vi "IMAQ-MWT GALVO XY Calibration (HOST).vi"() -> ()   [LabVIEW 2017]
uses:
  Modules/Common/Controls (HOST)/Image Size.ctl
  Modules/Common/Controls (HOST)/REF.ctl
  Modules/Common/Controls (HOST)/Image Queue Bundle.ctl
  Modules/Common/Controls (HOST)/Data to Disk Bundle.ctl
  Modules/Common/Controls (HOST)/File Name Prefix.ctl
  Modules/Common/Controls (HOST)/FPGA REF (MWT).ctl
  Modules/Common/Controls (HOST)/Experiment Mode.ctl
  Modules/Common/Controls (HOST)/Main States.ctl
  Modules/Common/Controls (HOST)/IMAQ Parameters.ctl
  Modules/Common/Controls (HOST)/File REF.ctl
  <vilib>/vision/Avi.llb/IMAQ AVI2 Refnum.ctl
  <vilib>/DAQmx/write.llb/DAQmx Write (Analog 1D DBL NChan 1Samp).vi
  <vilib>/Utility/error.llb/Error Cluster From Error Code.vi
  <vilib>/rvi/errors/niLvFpgaAdjustHostInterfaceError.vi
  <vilib>/FPGAPlugInAG/Dynamic/niLvFpga_Close_Dynamic.vi
  <vilib>/DAQmx/configure/timing.llb/DAQmx Timing (Sample Clock).vi
  <vilib>/DAQmx/miscellaneous.llb/DAQmx Fill In Error Info.vi
  <vilib>/rvi/interface/nirviReadWriteControl/nirviReadWriteControl.xnode
  <vilib>/rvi/interface/nirviCloseFPGA/nirviCloseFPGA.xnode
  NiFpgaLv.dll
  <vilib>/rvi/interface/Simulation/niFpgaSimulationCallBeginRW.vi
  <vilib>/vision/NI_Vision_Development_Module.lvlib
  <vilib>/Utility/file.llb/Write Delimited Spreadsheet (I64).vi
panel:
  in  "Calibrate":bool
  in  "Stop Button":bool
  out "GALVO Voltage":cluster{"X":dbl, "Y ":dbl}[](array[cluster]) {"X" format="%.3f"; "Y" format="%.3f"}
  out "Scan spots":cluster{"X":i32, "Y":i32}[](array[cluster])=[{"X"=200, "Y"=200}, {"X"=3000, "Y"=200}]
  in  "DAQmx Task Name":refnum<k21>="GALVO"
  out "IR SPOT (Measured)":cluster{"X":i32, "Y":i32}
  in  "Tab Control":enum32{"Setup"}(tab)
  in  "Image Size":T1={"Height"=3072, "Width"=3200}
  in  "Experiment Mode":T2
  in  "Pixel Intensity Range":cluster{"Low":u8, "High":u8}={"Low"=25, "High"=135}
  in  "Exp. Time (S)":dbl=120.0
  in  "Go":bool
  in  "Subtract BG":bool=TRUE
  in  "Replay Interval (ms)":u32=1000
  in  "Swap Bytes":bool
  out "Particle Reports (Pixels)":T3(array[cluster]) {"Orientation" format="%.2f"; "Dimensions"."Height" format="%.2f"; "Dimensions"."Width" format="%.2f"; "Center of Mass"."Y" format="%.2f"; "Center of Mass"."X" format="%.2f"; "Bounding Rect"."Bottom" format="%.2f"; "Bounding Rect"."Right" format="%.2f"; "Bounding Rect"."Top" format="%.2f"; "Bounding Rect"."Left" format="%.2f"; "Number of Holes" format="%.2f"; "Area" format="%.2f"}
  in  "Range":cluster{"Low":sgl, "High":sgl}={"Low"=3.0, "High"=255.0}
  in  "Selection Values":T5(array[cluster])=[{"Measurement Parameter"=18, "Range Lower Value"=50.0, "Range Upper Value"=1000.0, "Range"=FALSE, "Measurement Type"=FALSE}] {"Measurement Parameter" items=["Center of Mass X", "Center of Mass Y", "First Pixel X", "First Pixel Y", "Bounding Rect Left", "Bounding Rect Top", "Bounding Rect Right", "Bounding Rect Bottom", "Max Feret Diameter Start X", "Max Feret Diameter Start Y", "Max Feret Diameter End X", "Max Feret Diameter End Y", "Max Horiz. Segment Length Left", "Max Horiz. Segment Length Right", "Max Horiz. Segment Length Row", "-", "Bounding Rect Width", "Bounding Rect Height", "Bounding Rect Diagonal", "Perimeter", "Convex Hull Perimeter", "Holes' Perimeter", "Max Feret Diameter", "Equivalent Ellipse Major Axis", "Equivalent Ellipse Minor Axis", "Equivalent Ellipse Minor Axis (Feret)", "Equivalent Rect Long Side", "Equivalent Rect Short Side", "Equivalent Rect Diagonal", "Equivalent Rect Short Side (Feret)", "Average Horiz. Segment Length", "Average Vert. Segment Length", "Hydraulic Radius", "Waddel Disk Diameter", "-", "Area", "Holes' Area", "Particle & Holes' Area", "Convex Hull Area", "Image Area", "-", "Number of Holes", "Number of Horiz. Segments", "Number of Vert. Segments", "-", "Orientation", "Max Feret Diameter Orientation", "-", "% Area/Image Area", "% Area/(Particle & Holes' Area)", "Ratio of Equivalent Ellipse Axes", "Ratio of Equivalent Rect Sides", "-", "Elongation Factor", "Compactness Factor", "Heywood Circularity Factor", "Type Factor", "-", "Sum X", "Sum Y", "Sum XX", "Sum XY", "Sum YY", "Sum XXX", "Sum XXY", "Sum XYY", "Sum YYY", "-", "Moment of Inertia XX", "Moment of Inertia XY", "Moment of Inertia YY", "Moment of Inertia XXX", "Moment of Inertia XXY", "Moment of Inertia XYY", "Moment of Inertia YYY", "Norm. Moment of Inertia XX", "Norm. Moment of Inertia XY", "Norm. Moment of Inertia YY", "Norm. Moment of Inertia XXX", "Norm. Moment of Inertia XXY", "Norm. Moment of Inertia XYY", "Norm. Moment of Inertia YYY", "Hu Moment 1", "Hu Moment 2", "Hu Moment 3", "Hu Moment 4", "Hu Moment 5", "Hu Moment 6", "Hu Moment 7"]; "Range Lower Value" format="%.2f"; "Range Upper Value" format="%.2f"}
  out "Number of Particles":i32
  out "Frame #":u32
  out "Frame Rate":u32
  in  "GALVO Input Voltage (V)":T6 {"GALVO 4"."Y" format="%.3f"; "GALVO 4"."X" format="%.3f"; "GALVO 3"."Y" format="%.3f"; "GALVO 3"."X" format="%.3f"; "GALVO 2"."Y" format="%.3f"; "GALVO 2"."X" format="%.3f"; "GALVO 1"."Y" format="%.3f"; "GALVO 1"."X" format="%.3f"}
  in  "Start Location (Pixels)":cluster{"X":i32, "Y":i32}={"X"=300, "Y"=300}
  in  "End Location (Pixels)":cluster{"X":i32, "Y":i32}={"X"=2800, "Y"=2800}
  in  "STEP Size (Pixels)":i32=50
  in  "Y Reverse":bool=TRUE
  in  "X Reverse":bool
  in  "GALVO #":T7(ring)
  out "Elapsed Time (s)":dbl format="%.1f"
  out "Exp. Status":string="Camera Connected"
  out "REF":T8
  out "Command Q":refnum<queue>
  out "Display":T11(plugin-control)
  out "Stopped?":bool
  # "GALVO XY Auto Calibration"
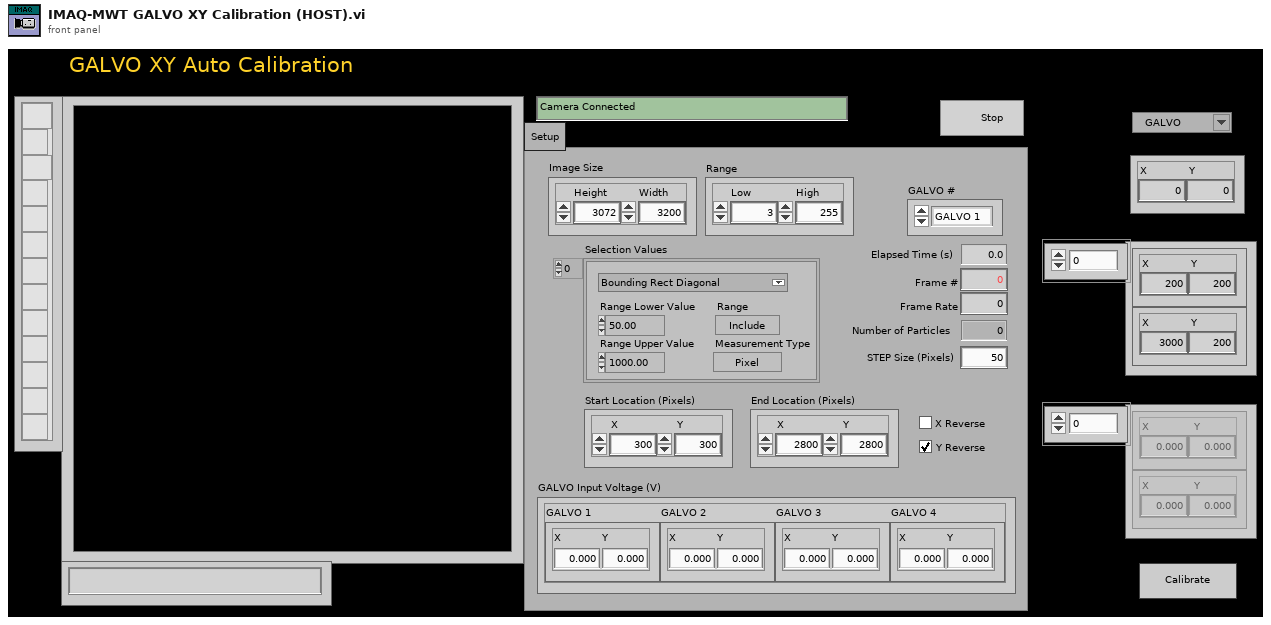
[diagram p1: front panel]
types:
  T1 = typedef "Image Size.ctl" = cluster{"Height":u16, "Width":u16}
  T2 = typedef "Experiment Mode.ctl" = enum16{"Live", "Replay"}
  T3 = cluster{"Area":dbl, "Number of Holes":dbl, "Bounding Rect":cluster{"Left":dbl, "Top":dbl, "Right":dbl, "Bottom":dbl}, "Center of Mass":cluster{"X":dbl, "Y":dbl}, "Orientation":dbl, "Dimensions":cluster{"Width":dbl, "Height":dbl}}[]
  T4 = typedef "Particle Parameters" = i32
  T5 = cluster{"Measurement Parameter":T4, "Range Lower Value":dbl, "Range Upper Value":dbl, "Range":bool, "Measurement Type":bool}[]
  T6 = cluster{"GALVO 1":cluster{"X":dbl, "Y ":dbl}, "GALVO 2":cluster{"X":dbl, "Y ":dbl}, "GALVO 3":cluster{"X":dbl, "Y ":dbl}, "GALVO 4":cluster{"X":dbl, "Y ":dbl}}
  T7 = enum16{"GALVO 1", "GALVO 2", "GALVO 3", "GALVO 4"}
  T8 = typedef "REF.ctl" = cluster{"Queue REF":T9, "FPGA REF (MWT)":T10}
  T9 = typedef "Image Queue Bundle.ctl" = cluster{"Disk Image":refnum<queue>, "Image Blocks":refnum<queue>, "Display Image":refnum<queue>, "BG Image":refnum<queue>, "Tag Image":refnum<queue>, "DLL Input":refnum<queue>, "DMD Input":refnum<queue>, "GALVO Input":refnum<queue>}
  T10 = typedef "FPGA REF (MWT).ctl" = refnum<k20>
  T11 = typedef "IMAQ Image.ctl" = refnum<image>
  T12 = enum8{"Enabled", "Disabled", "Disabled and Grayed Out"}
  T13 = typedef "Main States.ctl" = enum16{"Open FPGA", "Initialize", "Preview", "Acquire Images", "STOP"}
  T14 = typedef "IMAQ Parameters.ctl" = cluster{"File REF":T15, "Frame Data":cluster{"Width":u32, "Height":u32, "Frames Per Second":u32, "Codec":string}, "File Type":string, "Experiment Mode":T2, "Movie File Path":path}
  T15 = typedef "File REF.ctl" = cluster{"AVI REF":T16, "DBDE REF":refnum<file>}
  T16 = typedef "IMAQ AVI2 Refnum.ctl" = refnum<k20>
  T17 = typedef "Data to Disk Bundle.ctl" = cluster{"Frame Number":u64, "Time Stamp (us)":u64, "Image Data":u64[], "Contour":u32[], "Raw Image REF":refnum<data-value>, "Block Image REF":refnum<data-value>, "Block Box":u64[], "SPINE":u32[], "HT Angle":u64[], "Block Position":u64[], "SPINE Count":u32[], "Contour Count":u32[], "SPINE DIR":u8[]}
  T18 = cluster{"Area":dbl, "Number of Holes":dbl, "Bounding Rect":cluster{"Left":dbl, "Top":dbl, "Right":dbl, "Bottom":dbl}, "Center of Mass":cluster{"X":dbl, "Y":dbl}, "Orientation":dbl, "Dimensions":cluster{"Width":dbl, "Height":dbl}}
  T19 = cluster{"Left":dbl, "Top":dbl, "Right":dbl, "Bottom":dbl}
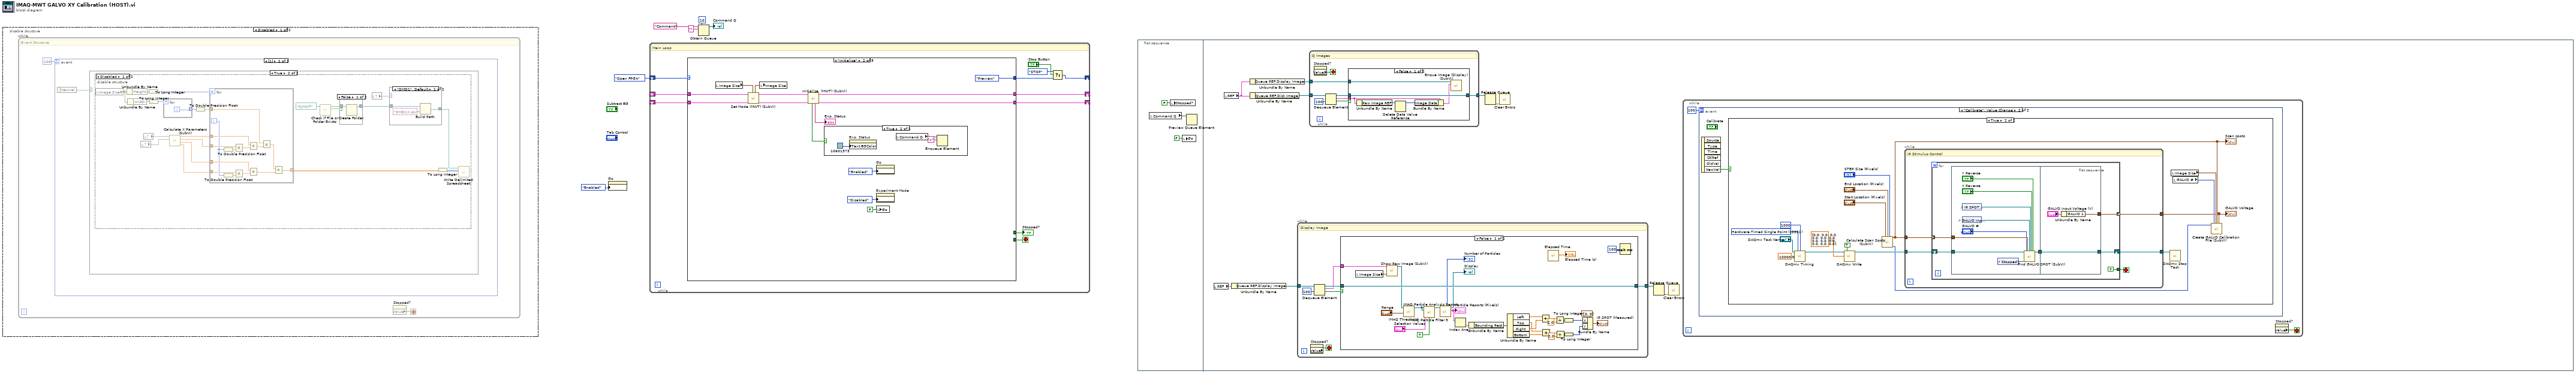
[diagram p0: block diagram]
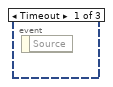
[diagram p2: hidden frame]
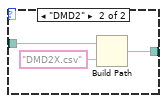
[diagram p5: hidden frame]
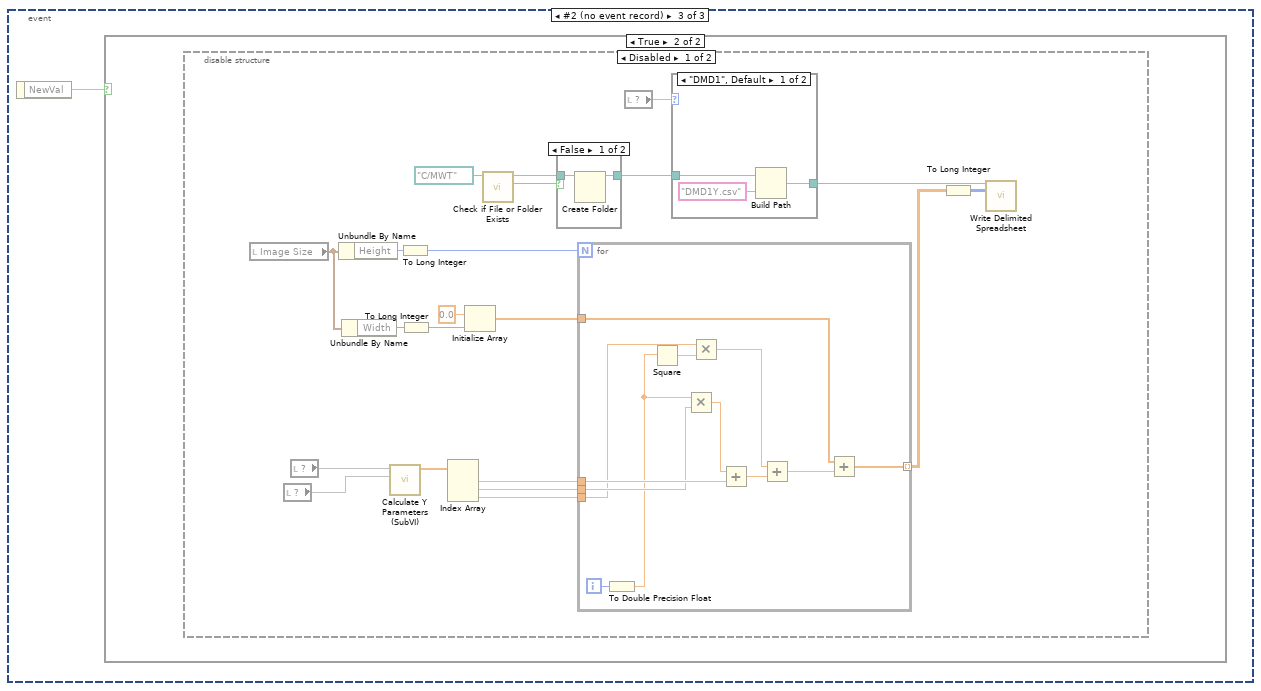
[diagram p7: hidden frame]
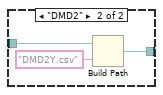
[diagram p10: hidden frame]
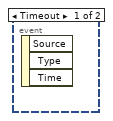
[diagram p13: hidden frame]
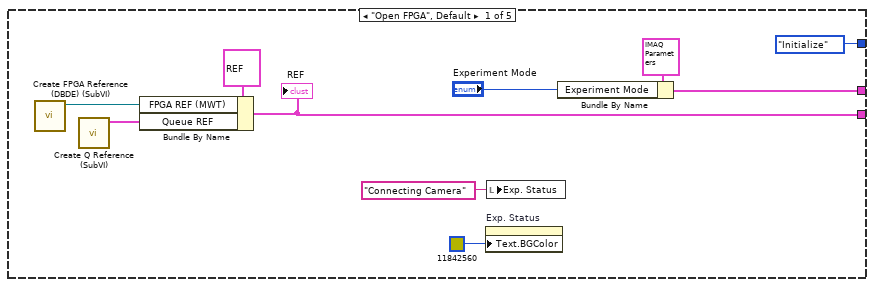
[diagram p17: hidden frame]
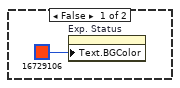
[diagram p18: hidden frame]
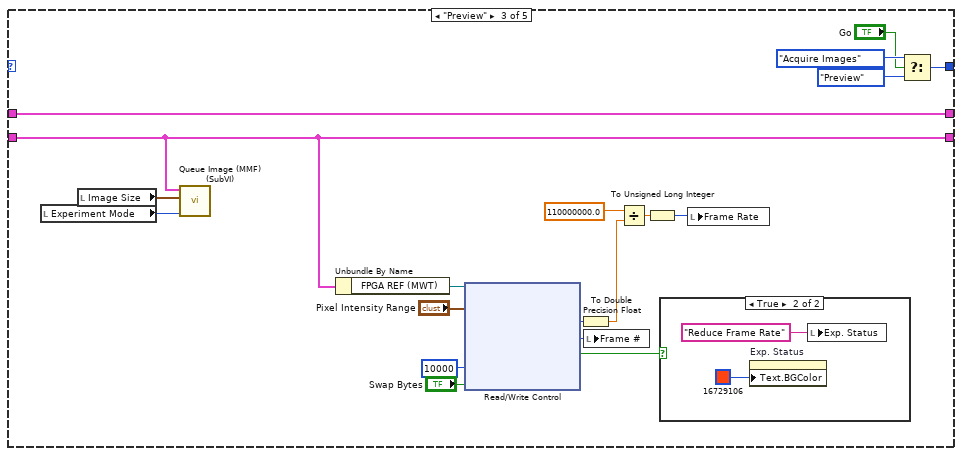
[diagram p19: hidden frame]
diagram:
  n1 = disable-structure shown="Disabled" {
    frame Disabled {
      n2 = while {
        stop <- w8 stop-if-true
        # "Event Structure"
        n3 = event shown="[1]" {
          selector: _ -> [_ _ _]
          dyn-events: _ -> [_ _ _]
          timeout: 100 -> [_ _ _]
          event Timeout {
            n4 = event-data() -> ()  [unwired: 1 in, 1 out]
          }
          event #1 (no event record) {
            n5 = event-data() -> ("NewVal"=w9)  [unwired: 1 in]
            n6 = case shown="True" w9 {
              frame False {
              }
              frame True {
                n7 = disable-structure shown="Disabled" {
                  frame Disabled {
                    n8 = local read "Image Size"() -> (w18:T1)
                    n9 = Unbundle By Name(w18) -> ("Height"=w30:u16)
                    n10 = Unbundle By Name(w18) -> ("Width"=w28:u16)
                    n11 = local read item#-1() -> (w24)
                    n12 = local read item#-1() -> (w23)
                    n13 = To Long Integer(number=w30) -> (32bit integer=w29:i32)
                    n14 = To Long Integer(number=w28) -> (32bit integer=w27:i32)
                    n15 = for {
                      N: w27 -> [_]
                      tunnel: [w40] -> w26 mode=indexing
                      i -> [w40]
                    }
                    n16 = call "Calculate X Parameters (SubVI).vi"("Camera"=w24, "DMD"=w23) -> ("Intercept Rate"=w19:dbl, "Intercept"=w20:dbl, "Slope Rate"=w21:dbl, "Slope"=w22:dbl)  [unwired: 6 in]
                    n17 = To Double Precision Float(number=w26) -> (double precision float=w25:dbl[])
                    n18 = for {
                      N: w29 -> [_]
                      tunnel: w25 -> [w49]
                      tunnel: w22 -> [w51]
                      tunnel: w21 -> [w54]
                      tunnel: w20 -> [w48]
                      tunnel: w19 -> [w45]
                      tunnel: [w41] -> w17 mode=indexing
                      i -> [w44]
                      n19 = To Double Precision Float(number=w44) -> (double precision float=w53:dbl)
                      n20 = To Double Precision Float(number=w44) -> (double precision float=w46:dbl)
                      n21 = Multiply(x=w54, y=w53) -> (x*y=w52:dbl)
                      n22 = Multiply(x=w45, y=w46) -> (x*y=w47:dbl)
                      n23 = Add(x=w51, y=w52) -> (x+y=w50:dbl)
                      n24 = Add(x=w48, y=w47) -> (x+y=w43:dbl)
                      n25 = Multiply(x=w49, y=w50) -> (x*y=w42:dbl[])
                      n26 = Add(x=w42, y=w43) -> (x+y=w41:dbl[])
                    }
                    n27 = call <vilib>:"Check if File or Folder Exists.vi"("path"=path "C:/MWT") -> ("file or folder exists?"=w14:bool, "dup path"=w13:path)  [unwired: 8 in, 1 out]
                    n28 = case shown="False" w14 {
                      tunnel: w13 -> [w32 w33]
                      tunnel: [w31 w33] -> w12
                      frame False {
                        n29 = Create Folder(path (use dialog)=w32) -> (created path=w31:path)  [unwired: 2 in, 2 out]
                      }
                      frame True {
                      }
                    }
                    n30 = local read item#-1() -> (w16)
                    n31 = case shown="\"DMD1\", Default" w16 {
                      tunnel: w12 -> [w36 w39]
                      tunnel: [w34 w37] -> w11
                      frame "DMD1", Default {
                        n32 = Build Path(base path=w36, name or relative path="DMD1X.csv") -> (appended path=w34:path)
                      }
                      frame "DMD2" {
                        n33 = Build Path(base path=w39, name or relative path="DMD2X.csv") -> (appended path=w37:path)
                      }
                    }
                    n34 = To Long Integer(number=w17) -> (32bit integer=w10:i32[][])
                    n35 = call-poly <vilib>:"Write Delimited Spreadsheet.vi"("file path (dialog if empty)"=w11, "2D data"=w10) -> ()  [unwired: 12 in, 2 out]
                  }
                  frame Enabled {
                  }
                }
              }
            }
          }
          event #2 (no event record) {
            n36 = event-data() -> ("NewVal"=w55)  [unwired: 1 in]
            n37 = case shown="True" w55 {
              frame False {
              }
              frame True {
                n38 = disable-structure shown="Disabled" {
                  frame Disabled {
                    n39 = local read "Image Size"() -> (w70:T1)
                    n40 = local read item#-1() -> (w74)
                    n41 = local read item#-1() -> (w75)
                    n42 = Unbundle By Name(w70) -> ("Height"=w71:u16)
                    n43 = Unbundle By Name(w70) -> ("Width"=w73:u16)
                    n44 = call "Calculate Y Parameters (SubVI).vi"("Camera"=w74, "DMD"=w75) -> ("Polynomial Coefficients"=w76:dbl[])  [unwired: 9 in]
                    n45 = To Long Integer(number=w71) -> (32bit integer=w72:i32)
                    n46 = To Long Integer(number=w73) -> (32bit integer=w59:i32)
                    n47 = Index Array(array=w76) -> (element #1=w61:dbl, element #2=w60:dbl, element #3=w56:dbl)  [unwired: 3 in]
                    n48 = Initialize Array(0.0 ("element"), w59) -> (w57:dbl[])
                    n49 = call <vilib>:"Check if File or Folder Exists.vi"("path"=path "C:/MWT") -> ("file or folder exists?"=w66:bool, "dup path"=w65:path)  [unwired: 8 in, 1 out]
                    n50 = case shown="False" w66 {
                      tunnel: w65 -> [w78 w79]
                      tunnel: [w77 w79] -> w64
                      frame False {
                        n51 = Create Folder(path (use dialog)=w78) -> (created path=w77:path)  [unwired: 2 in, 2 out]
                      }
                      frame True {
                      }
                    }
                    n52 = for {
                      N: w72 -> [_]
                      tunnel: [w87] -> w69 mode=indexing
                      tunnel: w61 -> [w95]
                      tunnel: w60 -> [w94]
                      tunnel: w57 -> [w86]
                      tunnel: w56 -> [w90]
                      i -> [w93]
                      n53 = To Double Precision Float(number=w93) -> (double precision float=w92:dbl)
                      n54 = Square(x=w92) -> (x^2=w91:dbl)
                      n55 = Multiply(x=w92, y=w94) -> (x*y=w97:dbl)
                      n56 = Multiply(x=w90, y=w91) -> (x*y=w88:dbl)
                      n57 = Add(x=w97, y=w95) -> (x+y=w96:dbl)
                      n58 = Add(x=w88, y=w96) -> (x+y=w89:dbl)
                      n59 = Add(x=w86, y=w89) -> (x+y=w87:dbl[])
                    }
                    n60 = local read item#-1() -> (w68)
                    n61 = case shown="\"DMD1\", Default" w68 {
                      tunnel: w64 -> [w80 w83]
                      tunnel: [w82 w85] -> w63
                      frame "DMD1", Default {
                        n62 = Build Path(base path=w80, name or relative path="DMD1Y.csv") -> (appended path=w82:path)
                      }
                      frame "DMD2" {
                        n63 = Build Path(base path=w83, name or relative path="DMD2Y.csv") -> (appended path=w85:path)
                      }
                    }
                    n64 = To Long Integer(number=w69) -> (32bit integer=w62:i32[][])
                    n65 = call-poly <vilib>:"Write Delimited Spreadsheet.vi"("file path (dialog if empty)"=w63, "2D data"=w62) -> ()  [unwired: 12 in, 2 out]
                  }
                  frame Enabled {
                  }
                }
              }
            }
          }
        }
        n66 = property on="Stopped?" class="Bool (strict)"() -> ("Value"=w8:bool)  [unwired: 2 in, 2 out]
      }
    }
    frame Enabled {
    }
  }
  n67 = property on="Go" class="Bool (strict)"("DisabledEnum"=T12."Enabled" ("Disabled")) -> ()  [unwired: 2 in, 2 out]
  n68 = while {
    shift-right: [w107] -> _
    shift-left: _ -> [w106]
    shift-right: [w98] -> _
    shift-left: Main_States."Open FPGA" -> [w108]
    shift-right: [w100] -> _
    shift-left: _ -> [w99]
    stop <- w104 stop-if-true
    # "Main Loop"
    n69 = case shown="\"Initialize\"" w108 {
      tunnel: [w115 w119 w140 w163 w193] -> w107
      tunnel: w106 -> [_ w120 w140 w163 w193]
      tunnel: [Main_States."Initialize" Main_States."Preview" w154 w182 Main_States."STOP"] -> w105
      tunnel: [_ _ _ _ w195] -> w104
      tunnel: [_ _ _ _ w195] -> w103
      tunnel: [w109 w124 w147 w166 w192] -> w100
      tunnel: w99 -> [_ w131 w147 w166 w192]
      frame "Open FPGA", Default {
        n70 = call "Create FPGA Reference (DBDE) (SubVI).vi"() -> ("FPGA REF (MWT)"=w117:T10)  [unwired: 11 in]
        n71 = call "Create Q Reference (SubVI).vi"() -> ("Image Queue"=w116:T9)  [unwired: 11 in]
        n72 = Bundle By Name(cluster=T8 {"Queue REF"={"Disk Image"=refnum, "Image Blocks"=refnum, "Display Image"=refnum, "BG Image"=refnum, "Tag Image"=refnum, "DLL Input"=refnum, "DMD Input"=refnum, "GALVO Input"=refnum}, "FPGA REF (MWT)"=refnum}, "FPGA REF (MWT)"=w117, "Queue REF"=w116) -> (w115:T8)
        "REF" <- w115
        n73 = property on="Exp. Status" class="Str"("Text.BGColor"=u32 11842560) -> ()  [unwired: 2 in, 2 out]
        n74 = local write "Exp. Status"("Connecting Camera" ("Exp. Status")) -> ()
        n75 = Bundle By Name(cluster=T14 {"File REF"={"AVI REF"=refnum, "DBDE REF"=refnum}, "Frame Data"={"Width"=0, "Height"=0, "Frames Per Second"=0, "Codec"=""}, "File Type"="", "Experiment Mode"=enum."Live", "Movie File Path"=path "D:/Movies Formatted on November 5th 2015/Clip (2) Formatted.raw"} ("Movie File Property"), "Experiment Mode"="Experiment Mode") -> (w109:T14)
      }
      frame "Initialize" {
        n76 = local read "Image Size"() -> (w122:T1)
        n77 = call "Set Mode (MWT) (SubVI).vi"("Image Size In"=w122, "REF IN"=w120, "Parameters In"=w131) -> ("REF OUT"=w123:T8, "Parameters Out"=w125:T14, "Image Size Out"=w121:T1)  [unwired: 6 in]
        n78 = local write "Image Size"(w121) -> ()
        n79 = call "Initialize  (MWT) (SubVI).vi"("REF IN"=w123, "Parameters In"=w125) -> ("REF OUT"=w119:T8, "Parameters Out"=w124:T14, "Exp. Status"=→"Exp. Status":string, "OK?"=w127:bool)  [unwired: 6 in]
        n80 = case shown="True" w127 {
          frame False {
            n81 = property on="Exp. Status" class="Str"("Text.BGColor"=u32 16729106) -> ()  [unwired: 2 in, 2 out]
          }
          frame True {
            n82 = property on="Exp. Status" class="Str"("Text.BGColor"=u32 10601373) -> ()  [unwired: 2 in, 2 out]
            n83 = local read "Command Q"() -> (w135:refnum<queue>)
            n84 = Enqueue Element(queue=w135, element="v") -> ()  [unwired: 2 in, 3 out]
          }
        }
        n85 = property on="Go" class="Bool (strict)"("DisabledEnum"=T12."Enabled" ("Disabled")) -> ()  [unwired: 2 in, 2 out]
        n86 = property on="Experiment Mode" class="Enum (strict)"("DisabledEnum"=T12."Disabled" ("Disabled")) -> ()  [unwired: 2 in, 2 out]
        n87 = local write "Go"(FALSE ("Go")) -> ()
      }
      frame "Preview" {
        n88 = local read "Experiment Mode"() -> (w138:T2)
        n89 = local read "Image Size"() -> (w144:T1)
        n90 = call "Queue Image (MMF) (SubVI).vi"("Experiment Mode"=w138, "Image Size"=w144, "Data Bundle"=w140) -> ()  [unwired: 9 in]
        n91 = Unbundle By Name(w140) -> ("FPGA REF (MWT)"=w150:T10)
        n92 = xnode "Read/Write Control"("FPGA VI Reference In"=w150, "Pixel Intensity"="Pixel Intensity Range", "Clock Cycles Limit"=u32 10000, "Swap Bytes"="Swap Bytes") -> ("Frame Interval"=w152:u32, "Frame #"=w143:u32, "DMA Timeout"=w142:bool)  [unwired: 1 in, 2 out]
        n93 = To Double Precision Float(number=w152) -> (double precision float=w151:dbl)
        n94 = local write "Frame #"(w143) -> ()
        n95 = Divide(x=110000000.0 ("y"), y=w151) -> (x/y=w148:dbl)
        n96 = To Unsigned Long Integer(number=w148) -> (unsigned 32bit integer=w146:u32)
        n97 = case shown="True" w142 {
          frame False {
          }
          frame True {
            n98 = property on="Exp. Status" class="Str"("Text.BGColor"=u32 16729106) -> ()  [unwired: 2 in, 2 out]
            n99 = local write "Exp. Status"("Reduce Frame Rate" ("Exp. Status")) -> ()
          }
        }
        n100 = local write "Frame Rate"(w146) -> ()
        n101 = Select(t=Main_States."Acquire Images", s="Go", f=Main_States."Preview") -> (s? t:f=w154:T13)
      }
      frame "Acquire Images" {
        n102 = local read "Experiment Mode"() -> (w161:T2)
        n103 = Unbundle By Name(w166) -> ("Experiment Mode"=w165:T2)
        n104 = call "Send Image to FPGA (SubVI).vi"("Data Bundle"=w163, "Parameters"=w166) -> ("TimeStamp"=w160:u64, "Frame Number"=w159:u64, "EOF"=w180:bool)  [unwired: 11 in]
        n105 = call "Queue Image (MMF) (SubVI).vi"("TimeStamp"=w160, "Frame Number"=w159, "Experiment Mode"=w161, "Image Size"="Image Size", "Data Bundle"=w163) -> ()  [unwired: 7 in]
        n106 = call "Get Elapsed Time (SubVI).vi"("Go"=TRUE, "Experiment Time (S)"="Exp. Time (S)") -> ("Done"=w171:bool, "Time Status"=w170:string)  [unwired: 8 in]
        n107 = Or(x=w171, y=w180) -> (x .or. y?=w172:bool)
        n108 = case shown="True" w180 {
          frame False {
          }
          frame True {
            n109 = One Button Dialog(message="End of Movie Reached") -> ()  [unwired: 1 in, 1 out]
          }
        }
        n110 = case shown="\"Replay\"" w165 {
          frame "Live", Default {
          }
          frame "Replay" {
            # "Limit image upload rate to 30 Hz"
            n111 = Wait (ms)(milliseconds to wait="Replay Interval (ms)") -> ()  [unwired: 1 out]
          }
        }
        n112 = local write "Exp. Status"(w170) -> ()
        n113 = local read "Pixel Intensity Range"() -> (w164:cluster{"Low":u8, "High":u8})
        n114 = Unbundle By Name(w163) -> ("FPGA REF (MWT)"=w177:T10)
        n115 = local read "Swap Bytes"() -> (w158:bool)
        n116 = xnode "Read/Write Control"("FPGA VI Reference In"=w177, "Pixel Intensity"=w164, "Significant Angle"=fxp<+,16,3> 0.0699462890625, "Swap Bytes"=w158) -> ("Frame Interval"=w179:u32, "Frame #"=→"Frame #":u32, "DMA Timeout"=w167:bool)  [unwired: 1 in, 2 out]
        n117 = case shown="True" w167 {
          frame False {
          }
          frame True {
            n118 = property on="Exp. Status" class="Str"("Text.BGColor"=u32 16729106) -> ()  [unwired: 2 in, 2 out]
            n119 = local write "Exp. Status"("Reduce Frame Rate" ("Exp. Status")) -> ()
          }
        }
        n120 = To Double Precision Float(number=w179) -> (double precision float=w178:dbl)
        n121 = Divide(x=110000000.0 ("y"), y=w178) -> (x/y=w174:dbl)
        n122 = To Unsigned Long Integer(number=w174) -> (unsigned 32bit integer=→"Frame Rate":u32)
        n123 = Select(t=Main_States."STOP", s=w172, f=Main_States."Acquire Images") -> (s? t:f=w182:T13)
      }
      frame "STOP" {
        w195 = TRUE
        n124 = Unbundle By Name(w193) -> ("FPGA REF (MWT)"=w194:T10)
        n125 = xnode "Close FPGA VI Reference"("FPGA VI Reference In"=w194) -> ("error out"=w189:errorcluster)  [unwired: 1 in]
        n126 = call <vilib>:"Clear Errors.vi"("error in (no error)"=w189) -> ()  [unwired: 5 in, 2 out]
        n127 = local write "Exp. Status"("Experiment Complete!" ("Exp. Status")) -> ()
        n128 = property on="Experiment Mode" class="Enum (strict)"("DisabledEnum"=T12."Enabled" ("Disabled")) -> ()  [unwired: 2 in, 2 out]
      }
    }
    "Stopped?" <- w103
    n129 = Select(t=Main_States."STOP", s="Stop Button", f=w105) -> (s? t:f=w98:T13)
  }
  n130 = Obtain Queue(max queue size (-1, unlimited)=10, name (unnamed)="Command", element data type="" ("name (unnamed)")) -> (queue out=→"Command Q":refnum<queue>)  [unwired: 2 in, 2 out]
  n131 = flat-sequence {
    frame #0 {
      n132 = local read "Command Q"() -> (w199:refnum<queue>)
      n133 = local write "Stopped?"(FALSE ("Stopped?")) -> ()
      n134 = local write "Go"(FALSE ("Go")) -> ()
      n135 = Preview Queue Element(queue=w199) -> ()  [unwired: 2 in, 4 out]
    }
    frame #1 {
      n136 = local read "REF"() -> (w207:T8)
      n137 = local read "REF"() -> (w202:T8)
      n138 = Unbundle By Name(w207) -> ("Queue REF.Display Image"=w206:refnum<queue>)
      n139 = Unbundle By Name(w202) -> ("Queue REF.Display Image"=w203:refnum<queue>)
      n140 = Unbundle By Name(w202) -> ("Queue REF.Disk Image"=w204:refnum<queue>)
      n141 = while {
        tunnel: [w270] -> w208
        tunnel: w206 -> [w269]
        stop <- w267 stop-if-true
        # "Display Image"
        n142 = property on="Stopped?" class="Bool (strict)"() -> ("Value"=w267:bool)  [unwired: 2 in, 2 out]
        n143 = Dequeue Element(queue=w269, timeout in ms (-1)=100) -> (queue out=w271:refnum<queue>, element=w268:T17, timed out?=w272:bool)  [unwired: 1 in, 1 out]
        n144 = case shown="False" w272 {
          tunnel: w271 -> [w303 w304]
          tunnel: [w303 w304] -> w270
          tunnel: w268 -> [w302 _]
          frame False {
            n145 = local read "Image Size"() -> (w300:T1)
            n146 = call "Show Raw Image (SubVI).vi"("Display Data"=w302, "Image Size"=w300) -> ("Image Out"=w299:T11)  [unwired: 17 in]
            n147 = call "IMAQ Threshold"("Range"="Range", "Image Src"=w299) -> ("Image Dst Out"=w298:T11)  [unwired: 8 in, 1 out]
            n148 = call "IMAQ Particle Filter 3"("Image Src"=w298, "Image Dst"=w298, "Selection Values"="Selection Values", "Fill Holes? (F)"=TRUE) -> ("Image Dst Out"=w296:T11)  [unwired: 9 in, 2 out]
            n149 = call "IMAQ Particle Analysis Report"("Image"=w296) -> ("Particle Reports (Pixels)"=w294:T3, "Image Out (duplicate)"=→"Display":T11, "Number of Particles"=→"Number of Particles":i32)  [unwired: 5 in, 3 out]
            "Particle Reports (Pixels)" <- w294
            n150 = Index Array(array=w294) -> (element=w293:T18)  [unwired: 1 in]
            n151 = Unbundle By Name(w293) -> ("Bounding Rect"=w292:T19)
            n152 = Unbundle By Name(w292) -> ("Left"=w291:dbl, "Top"=w284:dbl, "Right"=w290:dbl, "Bottom"=w285:dbl)
            n153 = Add(x=w291, y=w290) -> (x+y=w289:dbl)
            n154 = Add(x=w284, y=w285) -> (x+y=w286:dbl)
            n155 = call "Elapsed Time"() -> ("Elapsed Time (s)"=→"Elapsed Time (s)":dbl)  [unwired: 12 in, 7 out]
            n156 = Divide(x=w289, y=2.0) -> (x/y=w283:dbl)
            n157 = Divide(x=w286, y=2.0) -> (x/y=w282:dbl)
            n158 = To Long Integer(number=w283) -> (32bit integer=w278:i32)
            n159 = To Long Integer(number=w282) -> (32bit integer=w277:i32)
            n160 = Bundle By Name(cluster=cluster{"X":i32, "Y":i32} {"X"=0, "Y"=0}, "X"=w278, "Y"=w277) -> (→"IR SPOT (Measured)":cluster{"X":i32, "Y":i32})
            n161 = Wait (ms)(milliseconds to wait=u32 100) -> ()  [unwired: 1 out]
          }
          frame True {
          }
        }
      }
      n162 = while {
        tunnel: [w258] -> w205
        tunnel: w204 -> [w252]
        tunnel: w203 -> [w257]
        stop <- w253 stop-if-true
        # "Q Images"
        n163 = property on="Stopped?" class="Bool (strict)"() -> ("Value"=w253:bool)  [unwired: 2 in, 2 out]
        n164 = Dequeue Element(queue=w252, timeout in ms (-1)=100) -> (queue out=w255:refnum<queue>, element=w256:T17, timed out?=w254:bool)  [unwired: 1 in, 1 out]
        n165 = case shown="False" w254 {
          tunnel: w255 -> [w265 w266]
          tunnel: [w265 w266] -> w258
          tunnel: w257 -> [w264 _]
          tunnel: w256 -> [w262 _]
          frame False {
            n166 = Unbundle By Name(w262) -> ("Raw Image REF"=w263:refnum<data-value>)
            n167 = Delete Data Value Reference(data value reference=w263) -> (data value=w261:u64[])  [unwired: 1 in, 1 out]
            n168 = Bundle By Name(cluster=w262, "Image Data"=w261) -> (w260:T17)
            n169 = call "Enque Image (Display) (SubVI).vi"("Data Bundle"=w260, "Display Image REF"=w264) -> ()  [unwired: 10 in]
          }
          frame True {
          }
        }
      }
      n170 = Release Queue(queue=w205) -> (error out=w200:errorcluster)  [unwired: 2 in, 2 out]
      n171 = call <vilib>:"Clear Errors.vi"("error in (no error)"=w200) -> ()  [unwired: 5 in, 2 out]
      n172 = Release Queue(queue=w208) -> (error out=w201:errorcluster)  [unwired: 2 in, 2 out]
      n173 = call <vilib>:"Clear Errors.vi"("error in (no error)"=w201) -> ()  [unwired: 5 in, 2 out]
      n174 = while {
        stop <- w210 stop-if-true
        n175 = event shown="[1] \"Calibrate\": Value Change" {
          selector: _ -> [_ _]
          dyn-events: _ -> [_ _]
          timeout: 100 -> [_ _]
          event Timeout {
            n176 = event-data() -> ()  [unwired: 1 in, 3 out]
          }
          event "Calibrate": Value Change {
            n177 = event-data() -> ("NewVal"=w211:bool)  [unwired: 1 in, 5 out]
            n178 = case shown="True" w211 {
              frame False {
              }
              frame True {
                w226 = 12522 items=["Finite Samples"=10178, "Continuous Samples"=10123, "Hardware Timed Single Point"=12522] ("sample mode")
                n179 = call-poly <vilib>:"DAQmx Timing.vi"("task/channels in"="DAQmx Task Name", "sample mode"=w226, "samples per channel"=1000, "rate"=10000.0) -> ("task out"=w214:refnum<k21>)  [unwired: 10 in, 1 out]
                n180 = call-poly <vilib>:"DAQmx Write.vi"("task/channels in"=w214, "auto start"=TRUE, "data"=dbl[] [0.0, 0.0, 0.0, 0.0, 0.0, 0.0, 0.0, 0.0, 0.0, 0.0, 0.0, 0.0]) -> ("task out"=w213:refnum<k21>)  [unwired: 10 in, 2 out]
                n181 = call "Calculate Scan Spots (SubVI).vi"("Start Location (Pixels)"="Start Location (Pixels)", "End Location (Pixels)"="End Location (Pixels)", "STEP Size (Pixels)"="STEP Size (Pixels)") -> ("Scan Spots (Array)"=w218:cluster{"X":i32, "Y":i32}[], "Spot Count"=w216:i32[])  [unwired: 11 in]
                "Scan spots" <- w218
                n182 = while {
                  tunnel: [w233] -> w224
                  tunnel: w213 -> [w232]
                  tunnel: w218 -> [w230]
                  tunnel: [w229] -> w217
                  stop <- w231 stop-if-true
                  # "IR Stimulus Control"
                  n183 = for {
                    tunnel: w230 -> [w237] mode=indexing
                    shift-right: [w239] -> w233
                    shift-left: w232 -> [w238]
                    tunnel: [TRUE ("Stopped?")] -> w231
                    tunnel: [w234] -> w229 mode=indexing
                    n184 = flat-sequence {
                      tunnel: w238 -> [w247]
                      tunnel: w237 -> [w246]
                      tunnel: [w248] -> w235
                      tunnel: [w251] -> w239
                      tunnel: w235 -> [w251]
                      tunnel: [w249] -> w234
                      frame #0 {
                        n185 = control-ref of="IR SPOT (Measured)"() -> (w245:refnum<vi>)
                        n186 = control-ref of="GALVO Input Voltage (V)"() -> (w244:refnum<vi>)
                        n187 = control-ref of="Stopped?"() -> (w240:refnum<vi>)
                        n188 = call "Find GALVO SPOT (SubVI).vi"("REF In"=w247, "Stopped?"=w240, "GALVO #"="GALVO #", "IR SPOT (Target)"=w246, "GALVO Input Voltage (V)"=w244, "IR SPOT (Measured)"=w245, "X Reverse"="X Reverse", "Y Reverse"="Y Reverse") -> ("REF Out"=w248:refnum<k21>)  [unwired: 19 in]
                      }
                      frame #1 {
                        n189 = Unbundle By Name("GALVO Input Voltage (V)") -> ("GALVO 1"=w249:cluster{"X":dbl, "Y ":dbl})
                      }
                    }
                  }
                }
                "GALVO Voltage" <- w217
                n190 = call <vilib>:"DAQmx Stop Task.vi"("task/channels in"=w224) -> ()  [unwired: 13 in, 2 out]
                n191 = local read "Image Size"() -> (w220:T1)
                n192 = local read "GALVO #"() -> (w219:T7)
                n193 = call "Create GALVO Calibration File (SubVI).vi"("Spot Count"=w216, "GALVO #"=w219, "Image Size"=w220, "Scan Spots (Array)"=w218, "GALVO Voltage Inputs"=w217) -> ()  [unwired: 15 in]
              }
            }
          }
        }
        n194 = property on="Stopped?" class="Bool (strict)"() -> ("Value"=w210:bool)  [unwired: 2 in, 2 out]
      }
    }
  }
